vi "Lab Panel V6.00.vi"() -> ()   [LabVIEW 2017] (continued)
              n200 = call "sub vi-open serial port v1.vi"("Select COM port"=w207) -> ("Error"=→"Com Port Status":bool, "LOOPS"=→"Com setup loops":i32, "VISA Com out"=→"VISA Com out":refnum<visa-resource-name>)  [unwired: 12 in]
            }
            frame #1 {
              n201 = for {
                N: 3 -> [_]
                w258 = TRUE
                n202 = local read "Simulate"() -> (w220:bool)
                n203 = local write "Temp read loop"(0) -> ()
                n204 = case shown="True" w220 {
                  frame False {
                  }
                  frame True {
                    w260 = 20
                    n205 = local write "Ambient Volts"(2.92) -> ()
                    n206 = global write "Global display 3.vi" "Ref deg C"(w260) -> ()
                    n207 = local write "Ref deg C"(w260) -> ()
                  }
                }
                n208 = call "sub vi - GET ALL TEMP v7.vi"("LA01-EN"=w258, "simulate"=w220, "LA02-EN"=w258, "LA03-EN"=w258, "LA04-EN"=w258, "LA05-EN"=w258, "Gen Cal Value"=1) -> ("ID"=w219:T26, "LA01 TEMP"=w256:T27, "LA02 TEMP"=w249:T27, "LA03 TEMP"=w242:T27, "LA04 TEMP"=w235:T27, "LA05 TEMP"=w228:T27)  [unwired: 1 in, 2 out]
                n209 = local write "LAB05 TEMP"(w228) -> ()
                n210 = local write "LAB04 TEMP"(w235) -> ()
                n211 = Unbundle(w242) -> ("T1"=w239:dbl, "T2"=w238:dbl, "T3"=w237:dbl, "T4"=w236:dbl)  [unwired: 2 out]
                n212 = Unbundle(w256) -> ("T1"=w254:dbl, "T2"=w253:dbl, "T3"=w252:dbl, "T4"=w251:dbl)  [unwired: 2 out]
                n213 = Unbundle(w249) -> ("T1"=w246:dbl, "T2"=w245:dbl, "T3"=w244:dbl, "T4"=w243:dbl)  [unwired: 2 out]
                n214 = Unbundle(w235) -> ("T1"=w233:dbl, "T2"=w232:dbl, "T3"=w231:dbl, "T4"=w230:dbl)  [unwired: 2 out]
                n215 = Unbundle(w228) -> ("T1"=w226:dbl, "T2"=w225:dbl, "T3"=w224:dbl, "T4"=w223:dbl)  [unwired: 2 out]
                n216 = local write "LAB01 TEMP"(w256) -> ()
                n217 = local write "LAB02 TEMP"(w249) -> ()
                n218 = local write "LAB03 TEMP"(w242) -> ()
                n219 = Unbundle(w219) -> ("id1"=→"LAB01-TP":bool, "id2"=→"LAB02-TP":bool, "id3"=→"LAB03-TP":bool, "id4"=→"LAB04-TP":bool, "id5"=→"LAB05-TP":bool)
                n220 = local read "TEMP LA05"() -> (w227:T10)
                n221 = local read "TEMP LA04"() -> (w234:T10)
                n222 = local read "TEMP LA02"() -> (w248:T10)
                n223 = local read "TEMP LA03"() -> (w241:T10)
                n224 = local read "TEMP LA01"() -> (w255:T10)
                n225 = Bundle(cluster=w241, "TL-1"=w239, "TN-1"=w238, "TL-2"=w237, "TN-2"=w236) -> (w240:T10)  [unwired: 4 in]
                n226 = Bundle(cluster=w255, "TL-1"=w254, "TN-1"=w253, "TL-2"=w252, "TN-2"=w251) -> (w250:T10)  [unwired: 4 in]
                n227 = Bundle(cluster=w248, "TL-1"=w246, "TN-1"=w245, "TL-2"=w244, "TN-2"=w243) -> (w247:T10)  [unwired: 4 in]
                n228 = Bundle(cluster=w234, "TL-1"=w233, "TN-1"=w232, "TL-2"=w231, "TN-2"=w230) -> (w229:T10)  [unwired: 4 in]
                n229 = Bundle(cluster=w227, "TL-1"=w226, "TN-1"=w225, "TL-2"=w224, "TN-2"=w223) -> (w222:T10)  [unwired: 4 in]
                n230 = local write "TEMP LA03"(w240) -> ()
                n231 = local write "TEMP LA01"(w250) -> ()
                n232 = local write "TEMP LA02"(w247) -> ()
                n233 = local write "TEMP LA05"(w222) -> ()
                n234 = local write "TEMP LA04"(w229) -> ()
              }
            }
            frame #2 {
              w269 = 0
              n235 = local read "LAB01 TEMP"() -> (w271:T13)
              n236 = local read "SIG LAB01-2"() -> (w266:T2)
              n237 = Unbundle By Name(w271) -> ("T1 Live"=w264:dbl, "T1 Neut"=w263:dbl, "T2 Live"=w262:dbl, "T2 Neut"=w261:dbl)  [unwired: 2 out]
              n238 = local read "SIG LAB01-1"() -> (w268:T2)
              n239 = local read "TEMP LA01"() -> (w272:T10)
              n240 = Bundle By Name(cluster=w272, "TL-1"=w264, "TN-1"=w263, "TL-2"=w262, "TN-2"=w261, "TL -1COUNT"=w269, "TN-1 COUNT"=w269, "TL-2 COUNT"=w269, "TN-2 COUNT"=w269) -> (w270:T10)
              n241 = Bundle(cluster=w268, "Tmp Live"=w264, "Tmp Neut"=w263) -> (w267:T2)  [unwired: 3 in]
              n242 = Bundle(cluster=w266, "Tmp Live"=w262, "Tmp Neut"=w261) -> (w265:T2)  [unwired: 3 in]
              n243 = local write "SIG LAB01-2"(w265) -> ()
              n244 = local write "SIG LAB01-1"(w267) -> ()
              n245 = local write "TEMP LA01"(w270) -> ()
            }
            frame #3 {
              w281 = 0
              n246 = local read "LAB02 TEMP"() -> (w283:T13)
              n247 = Unbundle By Name(w283) -> ("T1 Live"=w276:dbl, "T1 Neut"=w275:dbl, "T2 Live"=w274:dbl, "T2 Neut"=w273:dbl)  [unwired: 2 out]
              n248 = local read "SIG LAB02-1"() -> (w280:T2)
              n249 = local read "SIG LAB02-2"() -> (w279:T2)
              n250 = local read "TEMP LA02"() -> (w284:T10)
              n251 = Bundle By Name(cluster=w284, "TL-1"=w276, "TN-1"=w275, "TL-2"=w274, "TN-2"=w273, "TL -1COUNT"=w281, "TN-1 COUNT"=w281, "TL-2 COUNT"=w281, "TN-2 COUNT"=w281) -> (w282:T10)
              n252 = Bundle(cluster=w279, "Tmp Live"=w274, "Tmp Neut"=w273) -> (w277:T2)  [unwired: 3 in]
              n253 = Bundle(cluster=w280, "Tmp Live"=w276, "Tmp Neut"=w275) -> (w278:T2)  [unwired: 3 in]
              n254 = local write "TEMP LA02"(w282) -> ()
              n255 = local write "SIG LAB02-1"(w278) -> ()
              n256 = local write "SIG LAB02-2"(w277) -> ()
            }
            frame #4 {
              w293 = 0
              n257 = local read "LAB03 TEMP"() -> (w295:T13)
              n258 = Unbundle By Name(w295) -> ("T1 Live"=w288:dbl, "T1 Neut"=w287:dbl, "T2 Live"=w286:dbl, "T2 Neut"=w285:dbl)  [unwired: 2 out]
              n259 = local read "SIG LAB03-1"() -> (w292:T2)
              n260 = local read "SIG LAB03-2"() -> (w291:T2)
              n261 = local read "TEMP LA03"() -> (w296:T10)
              n262 = Bundle By Name(cluster=w296, "TL-1"=w288, "TN-1"=w287, "TL-2"=w286, "TN-2"=w285, "TL -1COUNT"=w293, "TN-1 COUNT"=w293, "TL-2 COUNT"=w293, "TN-2 COUNT"=w293) -> (w294:T10)
              n263 = Bundle(cluster=w291, "Tmp Live"=w286, "Tmp Neut"=w285) -> (w289:T2)  [unwired: 3 in]
              n264 = Bundle(cluster=w292, "Tmp Live"=w288, "Tmp Neut"=w287) -> (w290:T2)  [unwired: 3 in]
              n265 = local write "TEMP LA03"(w294) -> ()
              n266 = local write "SIG LAB03-2"(w289) -> ()
              n267 = local write "SIG LAB03-1"(w290) -> ()
            }
            frame #5 {
              w305 = 0
              n268 = local read "LAB04 TEMP"() -> (w307:T13)
              n269 = Unbundle By Name(w307) -> ("T1 Live"=w300:dbl, "T1 Neut"=w299:dbl, "T2 Live"=w298:dbl, "T2 Neut"=w297:dbl)  [unwired: 2 out]
              n270 = local read "SIG LAB04-2"() -> (w303:T2)
              n271 = local read "SIG LAB04-1"() -> (w304:T2)
              n272 = local read "TEMP LA04"() -> (w308:T10)
              n273 = Bundle By Name(cluster=w308, "TL-1"=w300, "TN-1"=w299, "TL-2"=w298, "TN-2"=w297, "TL -1COUNT"=w305, "TN-1 COUNT"=w305, "TL-2 COUNT"=w305, "TN-2 COUNT"=w305) -> (w306:T10)
              n274 = Bundle(cluster=w303, "Tmp Live"=w298, "Tmp Neut"=w297) -> (w301:T2)  [unwired: 3 in]
              n275 = Bundle(cluster=w304, "Tmp Live"=w300, "Tmp Neut"=w299) -> (w302:T2)  [unwired: 3 in]
              n276 = local write "SIG LAB04-2"(w301) -> ()
              n277 = local write "TEMP LA04"(w306) -> ()
              n278 = local write "SIG LAB04-1"(w302) -> ()
            }
            frame #6 {
              w317 = 0
              n279 = local read "LAB05 TEMP"() -> (w319:T13)
              n280 = Unbundle By Name(w319) -> ("T1 Live"=w312:dbl, "T1 Neut"=w311:dbl, "T2 Live"=w310:dbl, "T2 Neut"=w309:dbl)  [unwired: 2 out]
              n281 = local read "SIG LAB05-2"() -> (w315:T2)
              n282 = local read "SIG LAB05-1"() -> (w316:T2)
              n283 = local read "TEMP LA05"() -> (w320:T10)
              n284 = Bundle By Name(cluster=w320, "TL-1"=w312, "TN-1"=w311, "TL-2"=w310, "TN-2"=w309, "TL -1COUNT"=w317, "TN-1 COUNT"=w317, "TL-2 COUNT"=w317, "TN-2 COUNT"=w317) -> (w318:T10)
              n285 = Bundle(cluster=w315, "Tmp Live"=w310, "Tmp Neut"=w309) -> (w313:T2)  [unwired: 3 in]
              n286 = Bundle(cluster=w316, "Tmp Live"=w312, "Tmp Neut"=w311) -> (w314:T2)  [unwired: 3 in]
              n287 = local write "SIG LAB05-2"(w313) -> ()
              n288 = local write "SIG LAB05-1"(w314) -> ()
              n289 = local write "TEMP LA05"(w318) -> ()
            }
          }
        }
        frame #11 {
          # "Create analog task"
          n290 = local read "Simulate"() -> (w321:bool)
          n291 = case shown="False" w321 {
            frame False {
              n292 = local read "SAMPLES"() -> (w324:dbl)
              n293 = local read "RATE (Hz)"() -> (w325:dbl)
              n294 = call "sub vi - AI USB4704 (3)  Create Task v4.vi"("Rate Hz"=w325, "Samples"=w324) -> ("TASK USB 0"=→"AI Task0":i32, "TASK USB 1"=→"AI Task1":i32, "TASK USB 2"=→"AI Task2":i32, "AI Task Er"=w322:bool)  [unwired: 9 in, 1 out]
              n295 = local write "Reset Error"(w322) -> ()
              "AI Task" <- TRUE
            }
            frame True {
            }
          }
        }
        frame #12 {
          # "Enable front panel, all settings done"
          n296 = property on="Tab Control 2" class="TabCtl (strict)"("DisabledEnum"=T17."Enabled" ("Disabled")) -> ()  [unwired: 2 in, 2 out]
          n297 = property on="Tab Control 2" class="TabCtl (strict)"("Value"=0) -> ()  [unwired: 2 in, 2 out]
        }
        frame #13 {
          n298 = property on="Tab Control 2" class="TabCtl (strict)"("Value"=0) -> ()  [unwired: 2 in, 2 out]
        }
      }
    }
    frame #2 {
      w332 = 250.0
      # "frames that only action on certain cycles, 13, 14, 15, 16, 19, 21"
      # "Main Loop"
      n299 = node-c288(w332) -> (w334:T19)  [unwired: 3 in]
      n300 = timed-loop {
        timing: w334 -> [_]
        timing-out: [_] -> w333
        tunnel: w332 -> [w335]
        i -> [w361]
        stop <- w336 stop-if-true
        n301 = node-c288() -> ()  [unwired: 1 in, 1 out]
        n302 = local read "Resets Done"() -> (w340:dbl)
        n303 = local read "SELECT LAB05-2"() -> (w341:T3)
        n304 = local read "SELECT LAB05-1"() -> (w342:T3)
        n305 = local read "SELECT LAB04-2"() -> (w343:T3)
        n306 = local read "SELECT LAB03-1"() -> (w346:T3)
        n307 = local read "SELECT LAB02-2"() -> (w347:T3)
        n308 = local read "SELECT LAB03-2"() -> (w345:T3)
        n309 = local read "SELECT LAB04-1"() -> (w344:T3)
        n310 = local read "SELECT LAB02-1"() -> (w348:T3)
        n311 = local read "run lab03-2"() -> (w355:bool)
        n312 = local read "run lab04-1"() -> (w354:bool)
        n313 = local read "run lab05-1"() -> (w352:bool)
        n314 = local read "run lab04-2"() -> (w353:bool)
        n315 = local read "run lab05-2"() -> (w351:bool)
        n316 = local read "run lab03-1"() -> (w356:bool)
        n317 = local read "run lab02-2"() -> (w357:bool)
        n318 = local read "SELECT LAB01-1"() -> (w350:T3)
        n319 = local read "SELECT LAB01-2"() -> (w349:T3)
        n320 = local read "run lab02-1"() -> (w358:bool)
        n321 = Greater?(x=w340, y=50) -> (0:w337:bool)
        n322 = Or(x=w337, y="stop") -> (x .or. y?=w336:bool)
        n323 = local read "run lab01-1"() -> (w360:bool)
        n324 = local read "run lab01-2"() -> (w359:bool)
        n325 = global write "Global display 1.vi" "stop disp"(w336) -> ()
        n326 = stacked-sequence {
          seq-local: [_ _ w447 _ _ _ _ _ _ _ _ _ _ _ _ _ _ _ _ _ _ _ _ _ _] -> [_ _ _ _ _ _ w2548 _ _ _ _ _ _ _ _ _ _ _ _ _ _ _ _ _ _]
          seq-local: [_ _ w446 _ _ _ _ _ _ _ _ _ _ _ _ _ _ _ _ _ _ _ _ _ _] -> [_ _ _ _ _ _ w2547 _ _ _ _ _ _ _ _ _ _ _ _ _ _ _ _ _ _]
          seq-local: [_ _ w433 _ _ _ _ _ _ _ _ _ _ _ _ _ _ _ _ _ _ _ _ _ _] -> [_ _ _ _ _ _ w2546 _ _ _ _ _ _ _ _ _ _ _ _ _ _ _ _ _ _]
          seq-local: [_ _ w432 _ _ _ _ _ _ _ _ _ _ _ _ _ _ _ _ _ _ _ _ _ _] -> [_ _ _ _ _ _ w2545 _ _ _ _ _ _ _ _ _ _ _ _ _ _ _ _ _ _]
          seq-local: [_ _ w431 _ _ _ _ _ _ _ _ _ _ _ _ _ _ _ _ _ _ _ _ _ _] -> [_ _ _ _ _ _ w2544 _ _ _ _ _ _ _ _ _ _ _ _ _ _ _ _ _ _]
          seq-local: [_ _ w430 _ _ _ _ _ _ _ _ _ _ _ _ _ _ _ _ _ _ _ _ _ _] -> [_ _ _ _ _ _ w2543 _ _ _ _ _ _ _ _ _ _ _ _ _ _ _ _ _ _]
          seq-local: [_ _ w429 _ _ _ _ _ _ _ _ _ _ _ _ _ _ _ _ _ _ _ _ _ _] -> [_ _ _ _ _ _ w2542 _ _ _ _ _ _ _ _ _ _ _ _ _ _ _ _ _ _]
          seq-local: [_ _ w428 _ _ _ _ _ _ _ _ _ _ _ _ _ _ _ _ _ _ _ _ _ _] -> [_ _ _ _ _ _ w2541 _ _ _ _ _ _ _ _ _ _ _ _ _ _ _ _ _ _]
          seq-local: [_ _ w427 _ _ _ _ _ _ _ _ _ _ _ _ _ _ _ _ _ _ _ _ _ _] -> [_ _ _ _ _ _ w2540 _ _ _ _ _ _ _ _ _ _ _ _ _ _ _ _ _ _]
          seq-local: [_ _ w426 _ _ _ _ _ _ _ _ _ _ _ _ _ _ _ _ _ _ _ _ _ _] -> [_ _ _ _ _ _ w2539 _ _ _ _ _ _ _ _ _ _ _ _ _ _ _ _ _ _]
          seq-local: [_ _ _ _ _ _ _ _ _ _ _ _ w3683 _ _ _ _ _ _ _ _ _ _ _ _] -> [_ _ _ _ _ _ _ _ _ _ _ _ _ w3715 _ _ _ _ _ _ _ _ _ _ _]
          tunnel: w360 -> [_ _ _ w463 w711 w2138 w2568 w2884 w3372 _ _ _ _ _ w3999 _ w4956 _ _ w5247 w5551 w5732 _ _ _]
          tunnel: w359 -> [_ _ _ w462 w709 w2137 w2567 w2885 w3371 _ _ _ _ _ w3998 _ w4954 _ _ w5246 w5550 w5730 _ _ _]
          tunnel: w358 -> [_ _ _ w461 w707 w2136 w2566 w2883 w3370 _ _ _ _ _ w3997 _ w4952 _ _ w5245 w5549 w5729 _ _ _]
          tunnel: w357 -> [_ _ _ w460 w705 w2135 w2565 w2882 w3369 _ _ _ _ _ w3996 _ w4950 _ _ w5244 w5548 w5728 _ _ _]
          tunnel: w356 -> [_ _ _ w459 w703 w2134 w2564 w2881 w3368 _ _ _ _ _ w3995 _ w4948 _ _ w5243 w5547 w5727 _ _ _]
          tunnel: w355 -> [_ _ _ w458 w701 w2133 w2563 w2880 w3367 _ _ _ _ _ w3994 _ w4946 _ _ w5242 w5546 w5726 _ _ _]
          tunnel: w354 -> [_ _ _ w457 w699 w2132 w2562 w2879 w3366 _ _ _ _ _ w3993 _ w4944 _ _ w5241 w5545 w5725 _ _ _]
          tunnel: w353 -> [_ _ _ w456 w697 w2131 w2561 w2878 w3365 _ _ _ _ _ w3992 _ w4942 _ _ w5240 w5544 w5724 _ _ _]
          tunnel: w352 -> [_ _ _ w455 w695 w2130 w2560 w2877 w3364 _ _ _ _ _ w3991 _ w4940 _ _ w5239 w5543 w5723 _ _ _]
          tunnel: w351 -> [_ _ _ w454 w693 w2129 w2559 w2876 w3363 _ _ _ _ _ w3990 _ w4938 _ _ w5238 w5542 w5722 _ _ _]
          tunnel: w350 -> [_ _ _ _ w710 w2128 w2558 _ _ _ _ _ _ _ _ _ w4958 _ _ _ _ _ w6193 _ _]
          tunnel: w349 -> [_ _ _ _ w708 w2127 w2557 _ _ _ _ _ _ _ _ _ w4953 _ _ _ _ _ w6192 _ _]
          tunnel: w348 -> [_ _ _ _ w706 w2126 w2556 _ _ _ _ _ _ _ _ _ w4951 _ _ _ _ _ w6191 _ _]
          tunnel: w347 -> [_ _ _ _ w704 w2125 w2555 _ _ _ _ _ _ _ _ _ w4949 _ _ _ _ _ w6190 _ _]
          tunnel: w346 -> [_ _ _ _ w702 w2124 w2554 _ _ _ _ _ _ _ _ _ w4947 _ _ _ _ _ w6189 _ _]
          tunnel: w345 -> [_ _ _ _ w700 w2123 w2553 _ _ _ _ _ _ _ _ _ w4945 _ _ _ _ _ w6188 _ _]
          tunnel: w344 -> [_ _ _ _ w698 w2122 w2552 _ _ _ _ _ _ _ _ _ w4943 _ _ _ _ _ w6187 _ _]
          tunnel: w343 -> [_ _ _ _ w696 w2121 w2551 _ _ _ _ _ _ _ _ _ w4941 _ _ _ _ _ w6186 _ _]
          tunnel: w342 -> [_ _ _ _ w694 w2120 w2550 _ _ _ _ _ _ _ _ _ w4939 _ _ _ _ _ w6185 _ _]
          tunnel: w341 -> [_ _ _ _ w692 w2119 w2549 _ _ _ _ _ _ _ _ _ w4937 _ _ _ _ _ w6184 _ _]
          tunnel: w337 -> [_ _ _ _ _ _ _ _ _ _ _ _ _ _ _ _ _ _ _ _ _ _ _ _ w6296]
          tunnel: w336 -> [_ _ _ _ _ _ _ _ _ _ _ _ _ _ _ _ _ _ _ _ _ _ _ _ w6295]
          tunnel: w335 -> [_ w383 _ _ _ _ _ _ _ _ _ _ _ _ _ _ _ _ _ _ _ _ _ _ _]
          frame #0 {
            n327 = local read "AI Task"() -> (w366:bool)
            n328 = global write "Global 1.vi" "RATE(Hz)"("RATE (Hz)") -> ()
            n329 = case shown="True" w366 {
              frame False {
              }
              frame True {
                n330 = local read "SAMPLES"() -> (w373:dbl)
                n331 = local read "AI Task2"() -> (w379:dbl)
                n332 = local read "AI Task1"() -> (w380:dbl)
                n333 = local read "AI Task0"() -> (w381:dbl)
                n334 = call "sub vi - AI USB4704 (3) v73.vi"("Task0"=w381, "Task1"=w380, "Task2"=w379, "SAMPLES"=w373) -> ("data 0"=→"AI data 0" →"AI Data 0":waveform(dbl)[], "data 1"=→"AI data 1" →"AI Data 1":waveform(dbl)[], "data 2"=→"AI data 2" →"AI Data 2":waveform(dbl)[], "loop time"=→"AI loop time":dbl, "error array"=→"AI Error":errorcluster[])  [unwired: 7 in]
              }
            }
            n335 = call <userlib>:"Periodic Trigger__ogtk.vi"("time (ms)"=u32 1000) -> ("Triggered"=w365:bool)  [unwired: 12 in, 2 out]
            n336 = case shown="True" w365 {
              frame False {
              }
              frame True {
                n337 = control-ref of="This VI"() -> (w372:refnum<vi>)
                n338 = invoke class="VI" method="FP.Get Image"(reference=w372) -> ("image data"=w371:T28)  [unwired: 5 in, 5 out]
                n339 = Build Path(base path="path to JPEG file", name or relative path="FP.jpg") -> (appended path=w368:path)
                n340 = call <vilib>:"Write JPEG File.vi"("image data"=w371, "path to JPEG file"=w368) -> ()  [unwired: 8 in, 2 out]
              }
            }
          }
          frame #1 {
            w390 = FALSE
            # "Loop time (s)"
            # "set up cycle control"
            n341 = local read "jig cycle"() -> (w394:dbl)
            n342 = local read "Amps Fail level"() -> (w388:dbl)
            n343 = local read "Simulate"() -> (w385:bool)
            n344 = Divide(x=w383, y=1000.0) -> (x/y=w382:dbl)
            n345 = Divide(x="JIG ON TIME (S)", y=w382) -> (x/y=→"on loops":dbl)
            n346 = Divide(x="JIG OFF TIME (S)", y=w382) -> (x/y=→"off loops":dbl)
            n347 = Increment(x=w394) -> (x+1=w393:dbl)
            n348 = local write "Simulate IND"(w385) -> ()
            n349 = global write "Global display 3.vi" "Amps Fail"(w388) -> ()
            n350 = local write "TEMP"(w390) -> ()
            n351 = local write "AI"(w390) -> ()
            n352 = local read "Network Directory"() -> (w387:path)
            n353 = local write "jig cycle"(w393) -> ()
            n354 = call "sub vi - check network dir v2.vi"("PATH"=w387) -> ("error"=w386:bool)  [unwired: 10 in]
            n355 = global write "Global display 3.vi" "network drive"(w386) -> ()
            n356 = event shown="[1] \"ADMIN\": Value Change" {
              selector: _ -> [_ _]
              dyn-events: _ -> [_ _]
              timeout: 10 -> [_ _]
              event Timeout {
                n357 = event-data() -> ()  [unwired: 1 in, 3 out]
              }
              event "ADMIN": Value Change {
                n358 = event-data() -> ()  [unwired: 1 in, 6 out]
                n359 = stacked-sequence {
                  seq-local: [_ w398 _] -> [_ _ w399]
                  frame #0 {
                    n360 = global write "Global 1.vi" "password"("9949") -> ()
                  }
                  frame #1 {
                    n361 = call "sub vi - password 1.vi"() -> ("RESULT"=w398:bool)  [unwired: 11 in]
                  }
                  frame #2 {
                    w401 = FALSE
                    n362 = property on="Tab Control 2" class="TabCtl (strict)"() -> ("Pages"=w405:refnum<vi>[])  [unwired: 2 in, 2 out]
                    n363 = Select(t=TRUE, s=w399, f=w401) -> (s? t:f=w400:bool)
                    n364 = Index Array(array=w405, index=8) -> (element=w403:refnum<vi>)
                    n365 = property class="Page"(reference=w403, "PageVis"=w400) -> ()  [unwired: 1 in, 2 out]
                    n366 = local write "ADMIN"(w401) -> ()
                  }
                }
              }
            }
            n367 = local write "network error"(w386) -> ()
          }
          frame #2 {
            w443 = 60.0
            # "Test Cycles"
            # "seconds"
            # "convert temperature rise minutes to cycles"
            n368 = local read "SET LAB05-2"() -> (w407:T5)
            n369 = local read "SET LAB05-1"() -> (w409:T5)
            n370 = local read "SET LAB04-2"() -> (w411:T5)
            n371 = local read "SET LAB01-1"() -> (w425:T6)
            n372 = local read "SET LAB01-2"() -> (w423:T5)
            n373 = local read "SET LAB02-2"() -> (w419:T5)
            n374 = local read "SET LAB04-1"() -> (w413:T5)
            n375 = local read "SET LAB03-1"() -> (w417:T5)
            n376 = local read "SET LAB03-2"() -> (w415:T5)
            n377 = local read "SET LAB02-1"() -> (w421:T5)
            n378 = local read "JIG OFF TIME (S)"() -> (w448:dbl)
            n379 = local read "JIG ON TIME (S)"() -> (w449:dbl)
            n380 = Unbundle By Name(w425) -> ("T-RISE mins"=w424:dbl)
            n381 = Unbundle(w407) -> ("T-RISE mins"=w406:dbl)  [unwired: 4 out]
            n382 = Unbundle(w409) -> ("T-RISE mins"=w408:dbl)  [unwired: 4 out]
            n383 = Unbundle(w411) -> ("T-RISE mins"=w410:dbl)  [unwired: 4 out]
            n384 = Unbundle(w423) -> ("T-RISE mins"=w422:dbl)  [unwired: 4 out]
            n385 = Unbundle(w421) -> ("T-RISE mins"=w420:dbl)  [unwired: 4 out]
            n386 = Unbundle(w413) -> ("T-RISE mins"=w412:dbl)  [unwired: 4 out]
            n387 = Unbundle(w419) -> ("T-RISE mins"=w418:dbl)  [unwired: 4 out]
            n388 = Unbundle(w415) -> ("T-RISE mins"=w414:dbl)  [unwired: 4 out]
            n389 = Unbundle(w417) -> ("T-RISE mins"=w416:dbl)  [unwired: 4 out]
            n390 = Add(x=w449, y=w448) -> (x+y=w442:dbl)
            n391 = Multiply(x=w443, y=w414) -> (x*y=w438:dbl)
            n392 = Multiply(x=w443, y=w412) -> (x*y=w437:dbl)
            n393 = Multiply(x=w443, y=w410) -> (x*y=w436:dbl)
            n394 = Multiply(x=w443, y=w408) -> (x*y=w435:dbl)
            n395 = Multiply(x=w443, y=w406) -> (x*y=w434:dbl)
            n396 = Multiply(x=w443, y=w422) -> (x*y=w444:dbl)
            n397 = Multiply(x=w443, y=w416) -> (x*y=w439:dbl)
            n398 = Multiply(x=w443, y=w424) -> (x*y=w445:dbl)
            n399 = Multiply(x=w443, y=w420) -> (x*y=w441:dbl)
            n400 = Multiply(x=w443, y=w418) -> (x*y=w440:dbl)
            n401 = Divide(x=w435, y=w442) -> (x/y=w427:dbl)
            n402 = Divide(x=w436, y=w442) -> (x/y=w428:dbl)
            n403 = Divide(x=w437, y=w442) -> (x/y=w429:dbl)
            n404 = Divide(x=w434, y=w442) -> (x/y=w426:dbl)
            n405 = Divide(x=w439, y=w442) -> (x/y=w431:dbl)
            n406 = Divide(x=w445, y=w442) -> (x/y=w447:dbl)
            n407 = Divide(x=w444, y=w442) -> (x/y=w446:dbl)
            n408 = Divide(x=w441, y=w442) -> (x/y=w433:dbl)
            n409 = Divide(x=w440, y=w442) -> (x/y=w432:dbl)
            n410 = Divide(x=w438, y=w442) -> (x/y=w430:dbl)
          }
          frame #3 {
            # "control cycle loops"
            n411 = local read "JIG OFF TIME (S)"() -> (w452:dbl)
            n412 = local read "JIG ON TIME (S)"() -> (w451:dbl)
            n413 = local read "on loops"() -> (w467:dbl)
            n414 = local read "off loops"() -> (w466:dbl)
            n415 = local read "jig cycle"() -> (w465:dbl)
            n416 = Add(x=w452, y=w451) -> (x+y=w450:dbl)
            n417 = Add(x=w467, y=w466) -> (x+y=w453:dbl)
            n418 = Greater Or Equal?(x=w465, y=w453) -> (x >= y?=w464:bool)
            n419 = case shown="True" w464 {
              tunnel: w463 -> [_ w501]
              tunnel: w462 -> [_ w500]
              tunnel: w461 -> [_ w499]
              tunnel: w460 -> [_ w498]
              tunnel: w459 -> [_ w497]
              tunnel: w458 -> [_ w496]
              tunnel: w457 -> [_ w495]
              tunnel: w456 -> [_ w494]
              tunnel: w455 -> [_ w493]
              tunnel: w454 -> [_ w492]
              tunnel: w450 -> [_ w491]
              frame False {
              }
              frame True {
                # "increment cycle value and convert cycles to minutes for temp rise"
                n420 = stacked-sequence {
                  frame #0 {
                    n421 = local read "Temp read loop"() -> (w504:dbl)
                    n422 = Increment(x=w504) -> (x+1=w503:dbl)
                    n423 = local write "Temp read loop"(w503) -> ()
                  }
                  frame #1 {
                    n424 = local read "Temp read loop"() -> (w505:dbl)
                    n425 = Greater?(x=w505, y=20) -> (0:w507:bool)
                    n426 = case shown="True" w507 {
                      frame False {
                      }
                      frame True {
                        n427 = local write "Temp read loop"(1) -> ()
                      }
                    }
                  }
                }
                n428 = local read "JIG RELAY CYCLES"() -> (w490:T9)
                n429 = local read "Temp read loop"() -> (→"Tp Up":dbl)
                n430 = Unbundle By Name(w490) -> ("LAB01-1"=w488:dbl, "LAB01-2"=w486:dbl, "LAB02-1"=w484:dbl, "LAB02-2"=w482:dbl, "LAB03-1"=w480:dbl, "LAB03-2"=w478:dbl, "LAB04-1"=w476:dbl, "LAB04-2"=w474:dbl, "LAB05-1"=w472:dbl, "LAB05-2"=w470:dbl)
                n431 = stacked-sequence {
                  tunnel: w501 -> [w519 _ _ _ _ _ _ _ _ _]
                  tunnel: w500 -> [_ w536 _ _ _ _ _ _ _ _]
                  tunnel: w499 -> [_ _ w553 _ _ _ _ _ _ _]
                  tunnel: w498 -> [_ _ _ w570 _ _ _ _ _ _]
                  tunnel: w497 -> [_ _ _ _ w587 _ _ _ _ _]
                  tunnel: w496 -> [_ _ _ _ _ w604 _ _ _ _]
                  tunnel: w495 -> [_ _ _ _ _ _ w621 _ _ _]
                  tunnel: w494 -> [_ _ _ _ _ _ _ w638 _ _]
                  tunnel: w493 -> [_ _ _ _ _ _ _ _ w655 _]
                  tunnel: w492 -> [_ _ _ _ _ _ _ _ _ w672]
                  tunnel: w491 -> [w516 w533 w550 w567 w584 w601 w618 w635 w652 w669]
                  tunnel: w488 -> [w510 _ _ _ _ _ _ _ _ _]
                  tunnel: [w509 _ _ _ _ _ _ _ _ _] -> w487
                  tunnel: w486 -> [_ w527 _ _ _ _ _ _ _ _]
                  tunnel: [_ w526 _ _ _ _ _ _ _ _] -> w485
                  tunnel: w484 -> [_ _ w544 _ _ _ _ _ _ _]
                  tunnel: [_ _ w543 _ _ _ _ _ _ _] -> w483
                  tunnel: w482 -> [_ _ _ w561 _ _ _ _ _ _]
                  tunnel: [_ _ _ w560 _ _ _ _ _ _] -> w481
                  tunnel: w480 -> [_ _ _ _ w578 _ _ _ _ _]
                  tunnel: [_ _ _ _ w577 _ _ _ _ _] -> w479
                  tunnel: w478 -> [_ _ _ _ _ w595 _ _ _ _]
                  tunnel: [_ _ _ _ _ w594 _ _ _ _] -> w477
                  tunnel: w476 -> [_ _ _ _ _ _ w612 _ _ _]
                  tunnel: [_ _ _ _ _ _ w611 _ _ _] -> w475
                  tunnel: w474 -> [_ _ _ _ _ _ _ w629 _ _]
                  tunnel: [_ _ _ _ _ _ _ w628 _ _] -> w473
                  tunnel: w472 -> [_ _ _ _ _ _ _ _ w646 _]
                  tunnel: [_ _ _ _ _ _ _ _ w645 _] -> w471
                  tunnel: w470 -> [_ _ _ _ _ _ _ _ _ w663]
                  tunnel: [_ _ _ _ _ _ _ _ _ w662] -> w469
                  frame #0 {
                    n432 = local read "DISP LAB01-1"() -> (w514:T4)
                    n433 = Unbundle By Name(w514) -> ("CYCLE"=w515:dbl)
                    n434 = case shown="True" w519 {
                      tunnel: w515 -> [w521 w525]
                      tunnel: [w521 w524] -> w513
                      tunnel: w510 -> [w520 w523]
                      tunnel: [w520 w522] -> w509
                      frame False {
                      }
                      frame True {
                        n435 = Increment(x=w523) -> (x+1=w522:dbl)
                        n436 = Increment(x=w525) -> (x+1=w524:dbl)
                      }
                    }
                    n437 = Multiply(x=w513, y=w516) -> (x*y=w517:dbl)
                    n438 = Divide(x=w517, y=60.0) -> (x/y=w512:dbl)
                    n439 = Bundle By Name(cluster=w514, "CYCLE"=w513, "MINS"=w512) -> (w511:T4)
                    n440 = local write "DISP LAB01-1"(w511) -> ()
                  }
                  frame #1 {
                    n441 = local read "DISP LAB01-2"() -> (w531:T4)
                    n442 = Unbundle By Name(w531) -> ("CYCLE"=w532:dbl)
                    n443 = case shown="True" w536 {
                      tunnel: w532 -> [w538 w542]
                      tunnel: [w538 w541] -> w529
                      tunnel: w527 -> [w537 w540]
                      tunnel: [w537 w539] -> w526
                      frame False {
                      }
                      frame True {
                        n444 = Increment(x=w540) -> (x+1=w539:dbl)
                        n445 = Increment(x=w542) -> (x+1=w541:dbl)
                      }
                    }
                    n446 = Multiply(x=w529, y=w533) -> (x*y=w534:dbl)
                    n447 = Divide(x=w534, y=60.0) -> (x/y=w528:dbl)
                    n448 = Bundle By Name(cluster=w531, "CYCLE"=w529, "MINS"=w528) -> (w530:T4)
                    n449 = local write "DISP LAB01-2"(w530) -> ()
                  }
                  frame #2 {
                    n450 = local read "DISP LAB02-1"() -> (w548:T4)
                    n451 = Unbundle By Name(w548) -> ("CYCLE"=w549:dbl)
                    n452 = case shown="True" w553 {
                      tunnel: [w555 w559] -> w546
                      tunnel: w549 -> [w555 w558]
                      tunnel: w544 -> [w554 w557]
                      tunnel: [w554 w556] -> w543
                      frame False {
                      }
                      frame True {
                        n453 = Increment(x=w557) -> (x+1=w556:dbl)
                        n454 = Increment(x=w558) -> (x+1=w559:dbl)
                      }
                    }
                    n455 = Multiply(x=w546, y=w550) -> (x*y=w551:dbl)
                    n456 = Divide(x=w551, y=60.0) -> (x/y=w545:dbl)
                    n457 = Bundle By Name(cluster=w548, "CYCLE"=w546, "MINS"=w545) -> (w547:T4)
                    n458 = local write "DISP LAB02-1"(w547) -> ()
                  }
                  frame #3 {
                    n459 = local read "DISP LAB02-2"() -> (w565:T4)
                    n460 = Unbundle By Name(w565) -> ("CYCLE"=w566:dbl)
                    n461 = case shown="True" w570 {
                      tunnel: [w572 w576] -> w564
                      tunnel: w566 -> [w572 w575]
                      tunnel: w561 -> [w571 w574]
                      tunnel: [w571 w573] -> w560
                      frame False {
                      }
                      frame True {
                        n462 = Increment(x=w574) -> (x+1=w573:dbl)
                        n463 = Increment(x=w575) -> (x+1=w576:dbl)
                      }
                    }
                    n464 = Multiply(x=w564, y=w567) -> (x*y=w568:dbl)
                    n465 = Divide(x=w568, y=60.0) -> (x/y=w563:dbl)
                    n466 = Bundle By Name(cluster=w565, "CYCLE"=w564, "MINS"=w563) -> (w562:T4)
                    n467 = local write "DISP LAB02-2"(w562) -> ()
                  }
                  frame #4 {
                    n468 = local read "DISP LAB03-1"() -> (w582:T4)
                    n469 = Unbundle(w582) -> ("CYCLE"=w583:dbl)  [unwired: 2 out]
                    n470 = case shown="True" w587 {
                      tunnel: [w589 w593] -> w579
                      tunnel: w583 -> [w589 w592]
                      tunnel: w578 -> [w588 w591]
                      tunnel: [w588 w590] -> w577
                      frame False {
                      }
                      frame True {
                        n471 = Increment(x=w591) -> (x+1=w590:dbl)
                        n472 = Increment(x=w592) -> (x+1=w593:dbl)
                      }
                    }
                    n473 = Multiply(x=w579, y=w584) -> (x*y=w585:dbl)
                    n474 = Divide(x=w585, y=60.0) -> (x/y=w580:dbl)
                    n475 = Bundle(cluster=w582, "CYCLE"=w579, "MINS"=w580) -> (w581:T4)  [unwired: 1 in]
                    n476 = local write "DISP LAB03-1"(w581) -> ()
                  }
                  frame #5 {
                    n477 = local read "DISP LAB03-2"() -> (w599:T4)
                    n478 = Unbundle(w599) -> ("CYCLE"=w600:dbl)  [unwired: 2 out]
                    n479 = case shown="True" w604 {
                      tunnel: [w606 w610] -> w598
                      tunnel: w600 -> [w606 w609]
                      tunnel: w595 -> [w605 w608]
                      tunnel: [w605 w607] -> w594
                      frame False {
                      }
                      frame True {
                        n480 = Increment(x=w608) -> (x+1=w607:dbl)
                        n481 = Increment(x=w609) -> (x+1=w610:dbl)
                      }
                    }
                    n482 = Multiply(x=w598, y=w601) -> (x*y=w602:dbl)
                    n483 = Divide(x=w602, y=60.0) -> (x/y=w597:dbl)
                    n484 = Bundle(cluster=w599, "CYCLE"=w598, "MINS"=w597) -> (w596:T4)  [unwired: 1 in]
                    n485 = local write "DISP LAB03-2"(w596) -> ()
                  }
                  frame #6 {
                    n486 = local read "DISP LAB04-1"() -> (w616:T4)
                    n487 = Unbundle(w616) -> ("CYCLE"=w617:dbl)  [unwired: 2 out]
                    n488 = case shown="True" w621 {
                      tunnel: [w623 w627] -> w614
                      tunnel: w617 -> [w623 w626]
                      tunnel: w612 -> [w622 w625]
                      tunnel: [w622 w624] -> w611
                      frame False {
                      }
                      frame True {
                        n489 = Increment(x=w625) -> (x+1=w624:dbl)
                        n490 = Increment(x=w626) -> (x+1=w627:dbl)
                      }
                    }
                    n491 = Multiply(x=w614, y=w618) -> (x*y=w619:dbl)
                    n492 = Divide(x=w619, y=60.0) -> (x/y=w613:dbl)
                    n493 = Bundle(cluster=w616, "CYCLE"=w614, "MINS"=w613) -> (w615:T4)  [unwired: 1 in]
                    n494 = local write "DISP LAB04-1"(w615) -> ()
                  }
                  frame #7 {
                    n495 = local read "DISP LAB04-2"() -> (w633:T4)
                    n496 = Unbundle(w633) -> ("CYCLE"=w634:dbl)  [unwired: 2 out]
                    n497 = case shown="True" w638 {
                      tunnel: [w640 w644] -> w631
                      tunnel: w634 -> [w640 w643]
                      tunnel: w629 -> [w639 w642]
                      tunnel: [w639 w641] -> w628
                      frame False {
                      }
                      frame True {
                        n498 = Increment(x=w642) -> (x+1=w641:dbl)
                        n499 = Increment(x=w643) -> (x+1=w644:dbl)
                      }
                    }
                    n500 = Multiply(x=w631, y=w635) -> (x*y=w637:dbl)
                    n501 = Divide(x=w637, y=60.0) -> (x/y=w630:dbl)
                    n502 = Bundle(cluster=w633, "CYCLE"=w631, "MINS"=w630) -> (w632:T4)  [unwired: 1 in]
                    n503 = local write "DISP LAB04-2"(w632) -> ()
                  }
                  frame #8 {
                    n504 = local read "DISP LAB05-1"() -> (w650:T4)
                    n505 = Unbundle(w650) -> ("CYCLE"=w651:dbl)  [unwired: 2 out]
                    n506 = case shown="True" w655 {
                      tunnel: [w657 w661] -> w648
                      tunnel: w651 -> [w657 w660]
                      tunnel: w646 -> [w656 w659]
                      tunnel: [w656 w658] -> w645
                      frame False {
                      }
                      frame True {
                        n507 = Increment(x=w659) -> (x+1=w658:dbl)
                        n508 = Increment(x=w660) -> (x+1=w661:dbl)
                      }
                    }
                    n509 = Multiply(x=w648, y=w652) -> (x*y=w653:dbl)
                    n510 = Divide(x=w653, y=60.0) -> (x/y=w647:dbl)
                    n511 = Bundle(cluster=w650, "CYCLE"=w648, "MINS"=w647) -> (w649:T4)  [unwired: 1 in]
                    n512 = local write "DISP LAB05-1"(w649) -> ()
                  }
                  frame #9 {
                    n513 = local read "DISP LAB05-2"() -> (w668:T4)
                    n514 = Unbundle(w668) -> ("CYCLE"=w667:dbl)  [unwired: 2 out]
                    n515 = case shown="True" w672 {
                      tunnel: [w674 w678] -> w666
                      tunnel: w667 -> [w674 w677]
                      tunnel: w663 -> [w673 w676]
                      tunnel: [w673 w675] -> w662
                      frame False {
                      }
                      frame True {
                        n516 = Increment(x=w676) -> (x+1=w675:dbl)
                        n517 = Increment(x=w677) -> (x+1=w678:dbl)
                      }
                    }
                    n518 = Multiply(x=w666, y=w669) -> (x*y=w670:dbl)
                    n519 = Divide(x=w670, y=60.0) -> (x/y=w665:dbl)
                    n520 = Bundle(cluster=w668, "CYCLE"=w666, "MINS"=w665) -> (w664:T4)  [unwired: 1 in]
                    n521 = local write "DISP LAB05-2"(w664) -> ()
                  }
                }
                n522 = local write "jig cycle"(0) -> ()
                n523 = Bundle By Name(cluster=w490, "LAB01-1"=w487, "LAB01-2"=w485, "LAB02-1"=w483, "LAB02-2"=w481, "LAB03-1"=w479, "LAB03-2"=w477, "LAB04-1"=w475, "LAB04-2"=w473, "LAB05-1"=w471, "LAB05-2"=w469) -> (w489:T9)
                n524 = local write "JIG RELAY CYCLES"(w489) -> ()
              }
            }
          }
          frame #4 {
            # "Note : Run lab0X-N variables are set which are written to digital I/O in frame 11"
            # "Why are these here?"
            # "START & STOP test RUN switch change, start test if true and stop test if false"
            n525 = Get Date/Time In Seconds() -> (seconds since 1Jan1904=w690:timestamp)
            n526 = local read "C drive data root dir"() -> (w683:path)
            n527 = Format Date/Time String(time format string (%c)="%b\\%a%d", seconds (now)=w690) -> (date/time string=w714:string)  [unwired: 1 in]
            n528 = Format Date/Time String(time format string (%c)="%H%M", seconds (now)=w690) -> (date/time string=w712:string)  [unwired: 1 in]
            n529 = Format Date/Time String(time format string (%c)="LabPanel%Y", seconds (now)=w690) -> (date/time string=w689:string)  [unwired: 1 in]
            n530 = Path To String(path=w683) -> (string=w686:string)
            n531 = global write "Global 1.vi" "C drive root path"(w683) -> ()
            n532 = local read "Ref deg C"() -> (w679:dbl)
            n533 = Concatenate Strings(w686, "\\") -> (w684:string)
            n534 = event shown="[10] \"RUN LAB05-2\": Value Change" {
              selector: _ -> [_ _ _ _ _ _ _ _ _ _ _]
              dyn-events: _ -> [_ _ _ _ _ _ _ _ _ _ _]
              timeout: 10 -> [_ _ _ _ _ _ _ _ _ _ _]
              tunnel: w684 -> [_ w727 w867 w1008 w1148 w1288 w1428 w1568 w1708 w1848 w1989]
              tunnel: w714 -> [_ w726 w866 w1007 w1147 w1287 w1427 w1567 w1707 w1847 w1988]
              tunnel: w712 -> [_ w724 w865 w1006 w1146 w1286 w1426 w1566 w1706 w1846 w1987]
              tunnel: w710 -> [_ w725 _ _ _ _ _ _ _ _ _]
              tunnel: w711 -> [_ _ _ _ _ _ _ _ _ _ _]
              tunnel: w709 -> [_ _ _ _ _ _ _ _ _ _ _]
              tunnel: w708 -> [_ _ w864 _ _ _ _ _ _ _ _]
              tunnel: w707 -> [_ _ _ _ _ _ _ _ _ _ _]
              tunnel: w706 -> [_ _ _ w1005 _ _ _ _ _ _ _]
              tunnel: w705 -> [_ _ _ _ _ _ _ _ _ _ _]
              tunnel: w704 -> [_ _ _ _ w1145 _ _ _ _ _ _]
              tunnel: w703 -> [_ _ _ _ _ _ _ _ _ _ _]
              tunnel: w702 -> [_ _ _ _ _ w1285 _ _ _ _ _]
              tunnel: w701 -> [_ _ _ _ _ _ _ _ _ _ _]
              tunnel: w700 -> [_ _ _ _ _ _ w1425 _ _ _ _]
              tunnel: w699 -> [_ _ _ _ _ _ _ _ _ _ _]
              tunnel: w698 -> [_ _ _ _ _ _ _ w1565 _ _ _]
              tunnel: w697 -> [_ _ _ _ _ _ _ _ _ _ _]
              tunnel: w696 -> [_ _ _ _ _ _ _ _ w1705 _ _]
              tunnel: w695 -> [_ _ _ _ _ _ _ _ _ _ _]
              tunnel: w694 -> [_ _ _ _ _ _ _ _ _ w1845 _]
              tunnel: w693 -> [_ _ _ _ _ _ _ _ _ _ _]
              tunnel: w692 -> [_ _ _ _ _ _ _ _ _ _ w1986]
              tunnel: w689 -> [_ w723 w863 w1004 w1144 w1284 w1424 w1564 w1704 w1844 w1985]
              tunnel: [_ w722 w862 w1003 w1143 w1283 w1423 w1563 w1703 w1843 w1984] -> w687
              tunnel: "RESET CYCLES TO ZERO?" -> [_ w721 w860 w1001 w1141 w1281 w1421 w1561 w1701 w1841 w1982]
              tunnel: "YES" -> [_ w720 w859 w1000 w1140 w1280 w1420 w1560 w1700 w1840 w1981]
              tunnel: "NO" -> [_ w719 w858 w999 w1139 w1279 w1419 w1559 w1699 w1839 w1980]
              tunnel: w679 -> [_ w716 w857 w997 w1138 w1278 w1418 w1558 w1698 w1838 w1978]
              event Timeout {
                n535 = event-data() -> ()  [unwired: 1 in, 3 out]
              }
              event "RUN LAB01-1": Value Change {
                n536 = event-data() -> ("NewVal"=w717:bool)  [unwired: 1 in, 5 out]
                n537 = local read "SIG LAB01-1"() -> (w718:T2)
                n538 = local write "run lab01-1"(w717) -> ()
                n539 = case shown="False" w717 {
                  tunnel: w727 -> [_ w765]
                  tunnel: w726 -> [_ w764]
                  tunnel: w725 -> [w729 w763]
                  tunnel: w724 -> [_ w762]
                  tunnel: w723 -> [_ w761]
                  tunnel: [w728 w760] -> w722
                  tunnel: w721 -> [_ w759]
                  tunnel: w720 -> [_ w758]
                  tunnel: w719 -> [_ w757]
                  tunnel: w718 -> [_ w756]
                  tunnel: w716 -> [_ w755]
                  frame False {
                    # "stop test"
                    n540 = stacked-sequence {
                      tunnel: w729 -> [_ w741 _]
                      tunnel: [_ w733 _] -> w728
                      frame #0 {
                        n541 = local read "DISP LAB01-1"() -> (w732:T4)
                        n542 = Bundle(cluster=w732, "STATUS"="STOP") -> (w730:T4)  [unwired: 2 in]
                        n543 = local write "DISP LAB01-1"(w730) -> ()
                      }
                      frame #1 {
                        n544 = local read "DISP LAB01-1"() -> (w740:T4)
                        n545 = Unbundle(w740) -> ("CYCLE"=w738:dbl, "MINS"=w739:dbl)  [unwired: 1 out]
                        n546 = case shown="\"CYCLE TEST\"" w741 {
                          tunnel: w739 -> [_ _ w748]
                          tunnel: w738 -> [w746 w747 _]
                          tunnel: [w746 w747 w748] -> w737
                          frame "CHART TEST", Default {
                          }
                          frame "CYCLE TEST" {
                          }
                          frame "T-RISE TEST" {
                          }
                        }
                        n547 = local read "TDMS LAB01-1"() -> (w745:refnum<k34>)
                        n548 = Build Array("STOPPED") -> (w742:string[])
                        n549 = Build Array(w737) -> (w736:dbl[])
                        n550 = TDMS Write(0:w745, 5:"TEST RESULT", 7:w742, 9:w736) -> (4:w734:refnum<k34>, 15:w735:errorcluster)  [unwired: 2 in, 2 out]
                        n551 = TDMS Close(8:w735, 11:w734) -> (0:w733:errorcluster)  [unwired: 1 out]
                      }
                      frame #2 {
                        n552 = stacked-sequence {
                          tunnel: "LAB01-1" -> [w751 w753]
                          frame #0 {
                            n553 = call "sub vi - defrag tdms v1.vi"("panel id"=w751) -> ("error out"=w750:errorcluster)  [unwired: 10 in]
                            n554 = local write "data file error"(w750) -> ()
                          }
                          frame #1 {
                            n555 = call "Save data file (stop) v3.vi"("panel id"=w753) -> ("network file save error"=w752:errorcluster)  [unwired: 9 in, 1 out]
                            n556 = local write "RESULT LAB01-1"(FALSE) -> ()
                            n557 = local write "data file error"(w752) -> ()
                          }
                        }
                      }
                    }
                  }
                  frame True {
                    n558 = stacked-sequence {
                      seq-local: [w767 _] -> [_ w771]
                      tunnel: w765 -> [_ w781]
                      tunnel: w764 -> [_ w780]
                      tunnel: w763 -> [_ w779]
                      tunnel: w762 -> [_ w778]
                      tunnel: w761 -> [_ w777]
                      tunnel: [_ w776] -> w760
                      tunnel: w759 -> [_ w775]
                      tunnel: w758 -> [_ w774]
                      tunnel: w757 -> [_ w773]
                      tunnel: w756 -> [w769 w772]
                      tunnel: w755 -> [_ w770]
                      frame #0 {
                        n559 = Unbundle(w769) -> ("AMPS"=w768:dbl)  [unwired: 4 out]
                        n560 = call "Check For Amps on v1.vi"("ID"="LAB01-1", "amps"=w768) -> ("amps"=w767:bool)  [unwired: 9 in]
                      }
                      frame #1 {
                        n561 = case shown="True" w771 {
                          tunnel: w781 -> [_ w794]
                          tunnel: w780 -> [_ w793]
                          tunnel: w779 -> [_ w792]
                          tunnel: w778 -> [_ w791]
                          tunnel: w777 -> [_ w790]
                          tunnel: [errorcluster {"status"=FALSE, "code"=0, "source"=""} ("error out") w789] -> w776
                          tunnel: w775 -> [_ w788]
                          tunnel: w774 -> [_ w787]
                          tunnel: w773 -> [_ w786]
                          tunnel: w772 -> [_ w785]
                          tunnel: w770 -> [_ w784]
                          frame False {
                            w782 = FALSE
                            n562 = local write "RUN LAB01-1"(w782) -> ()
                            n563 = local write "run lab01-1"(w782) -> ()
                          }
                          frame True {
                            n564 = stacked-sequence {
                              seq-local: [w795 _ _ _ _] -> [_ w816 _ _ _]
                              tunnel: w794 -> [w800 _ _ _ _]
                              tunnel: w793 -> [w796 _ _ _ _]
                              tunnel: w792 -> [w810 _ _ _ _]
                              tunnel: w791 -> [w803 _ _ _ _]
                              tunnel: w790 -> [w798 _ _ _ _]
                              tunnel: [_ w817 _ _ _] -> w789
                              tunnel: w788 -> [_ _ _ w838 _]
                              tunnel: w787 -> [_ _ _ w848 _]
                              tunnel: w786 -> [_ _ _ w847 _]
                              tunnel: w785 -> [_ _ _ _ _]
                              tunnel: w784 -> [_ _ _ _ w854]
                              frame #0 {
                                w797 = "\\"
                                n565 = case shown="\"CHART TEST\", Default" w810 {
                                tunnel: ["L01-1-CHART TEST-" "L01-1-CYCLE TEST-" "L01-1-T-RISE TEST-"] -> w806
                                frame "CHART TEST", Default {
                                }
                                frame "CYCLE TEST" {
                                }
                                frame "T-RISE TEST" {
                                }
                                }
                                n566 = local read "SET LAB01-1"() -> (w805:T6)
                                n567 = Unbundle By Name(w805) -> ("DESCRIPTION"=w804:string)
                                n568 = Concatenate Strings(w800, "\\", w798, w797, w796, w797) -> (w807:string)
                                n569 = String To Path(string=w807) -> (path=w809:path)
                                n570 = Concatenate Strings(w807, w806, w804, "-", w803, ".tdms") -> (w795:string)
                                n571 = Create Folder(path (use dialog)=w809) -> (error out=w808:errorcluster)  [unwired: 2 in, 2 out]
                                n572 = call <vilib>:"Clear Errors.vi"("error in (no error)"=w808) -> ()  [unwired: 5 in, 2 out]
                                n573 = global write "Global 1.vi" "LAB01-1 FILE"(w795) -> ()
                              }
                              frame #1 {
                                (unwired) FALSE
                                n574 = String To Path(string=w816) -> (path=w814:path)
                                n575 = TDMS Open(6:FALSE, 10:T22."create or replace" ("operation (0:open)"), 11:w814) -> (0:w817:errorcluster, 3:→"TDMS LAB01-1":refnum<k34>)  [unwired: 4 in]
                              }
                              frame #2 {
                                n576 = local read "TDMS LAB01-1"() -> (w836:refnum<k34>)
                                n577 = local read "SET LAB01-1"() -> (w825:T6)
                                n578 = Build Array("Testers Name", "Description", "Set Test Cycles", "T-Rise minutes", "T-Rise Deg C") -> (w826:string[])
                                n579 = Unbundle(w825) -> ("NAME"=w824:string, "DESCRIPTION"=w823:string, "CYCLES"=w822:dbl, "T-RISE mins"=w821:dbl, "T-RISE deg C"=w820:dbl)
                                n580 = Number To Decimal String(number=w822) -> (decimal integer string=w835:string)  [unwired: 1 in]
                                n581 = Number To Decimal String(number=w821) -> (decimal integer string=w834:string)  [unwired: 1 in]
                                n582 = Number To Decimal String(number=w820) -> (decimal integer string=w833:string)  [unwired: 1 in]
                                n583 = Build Array(w824, w823, w835, w834, w833) -> (w832:string[])
                                n584 = TDMS Set Properties(5:w832, 7:w826, 11:w836) -> ()  [unwired: 3 in, 4 out]
                              }
                              frame #3 {
                                n585 = local read "DISP LAB01-1"() -> (w846:T4)
                                n586 = Concatenate Strings("LAB01-1  ", w838) -> (w837:string)
                                n587 = Two Button Dialog(message=w837, 1:w847, 2:w848) -> (T button?=w840:bool)
                                n588 = case shown="True" w840 {
                                tunnel: w846 -> [w851 w852]
                                tunnel: [w851 w852] -> w845
                                tunnel: [w850 w853] -> w844
                                tunnel: [w849 w853] -> w843
                                frame False {
                                n589 = Unbundle(w851) -> ("CYCLE"=w850:dbl, "MINS"=w849:dbl)  [unwired: 1 out]
                                }
                                frame True {
                                w853 = 0.0
                                }
                                }
                                n590 = Bundle(cluster=w845, "CYCLE"=w844, "MINS"=w843, "STATUS"="RUN") -> (w842:T4)
                                n591 = local write "DISP LAB01-1"(w842) -> ()
                              }
                              frame #4 {
                                n592 = local read "TEMP START LAB01-1"() -> (w856:cluster{"TL":dbl, "TN":dbl})
